vi "RT_create_network_stream_writers.vi"(8 "error in (no error)":errorcluster) -> (0 "error out":errorcluster, 2 "Count Writer":refnum<k21>, 3 "Analog Writer":refnum<k21>)   [LabVIEW 2020]
uses:
  <vilib>/dex/Stream Element Allocation Mode.ctl
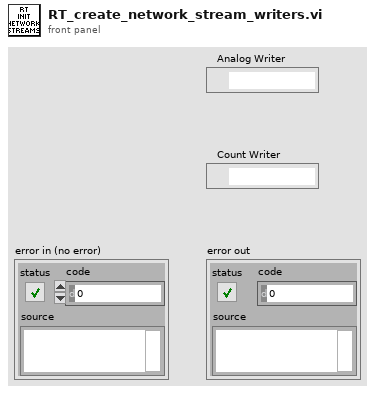
[diagram p1: front panel]
types:
  T1 = typedef "Stream Element Allocation Mode.ctl" = u32
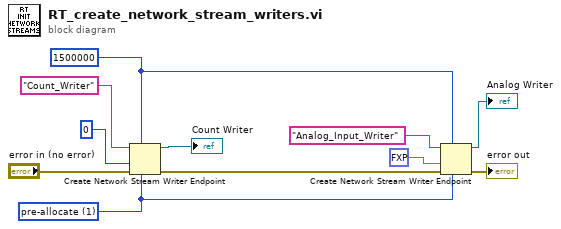
[diagram p0: block diagram]
diagram:
  w1 = T1 1 items=["allocate as needed", "pre-allocate"] ("element allocation mode")
  w2 = 1500000 ("writer buffer size")
  n1 = Create Network Stream Writer Endpoint(6:w1, 7:w2, 8:"error in (no error)", 9:0, 11:"Count_Writer" ("writer name")) -> (0:w8:errorcluster, 3:→"Count Writer":refnum<k21>)  [unwired: 2 in]
  n2 = Create Network Stream Writer Endpoint(6:w1, 7:w2, 8:w8, 9:fxp<+/-,17,5> 0.0, 11:"Analog_Input_Writer" ("writer name")) -> (0:→"error out":errorcluster, 3:→"Analog Writer":refnum<k21>)  [unwired: 2 in]
